vi "RLCar_joystick.vi"() -> ()   [LabVIEW 2021]
uses:
  Ctrl/joystick cfg.ctl
  Ctrl/joy-axis.ctl
  Ctrl/cmd_common.ctl
  <vilib>/Instr/_visa.llb/VISA Configure Serial Port (Instr).vi
  Log/_common_log/logfile-name.vi
panel:
  in  "Joystick cfg 2":T1={"steer limit"={"scale"=13.0, "offset"=32.0}, "speed limit"={"min"=10.0, "max"=161.0}, "Axis"={"man"=0.0, "auto"=0.0, "angular"=enum."Z rotation", "linear"=enum."X axis", "linear inv"=TRUE, "ang inv"=FALSE}} {"speed limit"."max" min=0.0 max=254.0 step=1.0}
  out "log path":string="C:\\RLmodel_cfg\\Log\\RLRobot\\2024-01-17-957\\Log_20240117-0957.txt"
  out "pos str":string="0"
  out "sp":dbl
  out "st":dbl=25.0 format="%.1f"
  out "val check":bool
  out "cmd_vel":cluster{dbl, dbl} {"?" format="%#.1f"; "?" format="%.1f"}
  out "n":i32=110
  out "XY Graph":cluster{cluster{"X":dbl, "Y":dbl}[]}[](graph)
  out "error out":errorcluster={"status"=FALSE, "code"=1073676294, "source"="VISA Read in RLCar_joystick.vi"}
  in  "port":refnum<visa-resource-name>="COM20"
  in  "rate":u32=115200
  out "Status":string
  out "String":string="sp=0,st=25,dir=b,light=1,pos=0,&\r\n"
  out "write buffer":string="0,25,b,1,RLCar kit ., &"
  in  "Led":bool=TRUE
  in  "msg":string="RLCar kit "
  in  "Write":bool=TRUE
  out "seriai buff":u32(graph)=34
  out "N":i32=221
  out "read buffer":string="sp=0,st=25,dir=b,light=1,pos=0,&\r\n"
  out "read buffer 2":string="sp=0,st=25,dir=b,light=1,pos=0,&\r\n"
  out "seriai R feedback":i32(graph)
  out "speed":dbl(graph)
  out "pos int":i32
  in  "dt":u32=50
  out "Recovery":i32
  in  "stop":bool=TRUE
  # "RLCar joystick controll"
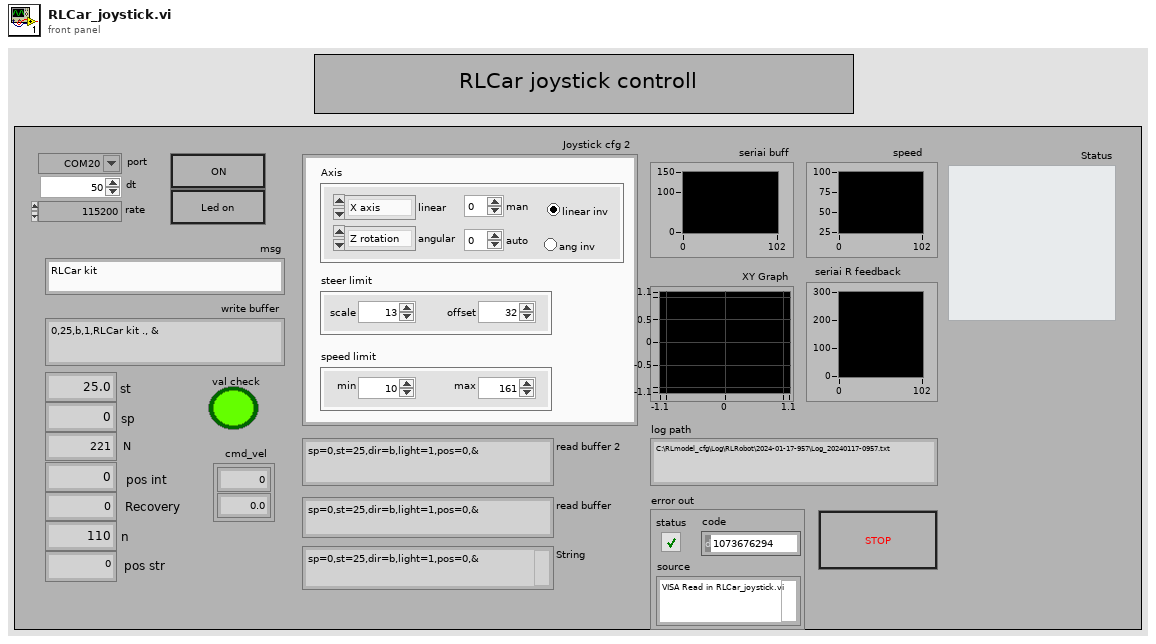
[diagram p1: front panel]
types:
  T1 = typedef "joystick cfg.ctl" = cluster{"steer limit":cluster{"scale":dbl, "offset":dbl}, "speed limit":cluster{"min":dbl, "max":dbl}, "Axis":cluster{"man":dbl, "auto":dbl, "angular":T2, "linear":T2, "linear inv":bool, "ang inv":bool}}
  T2 = typedef "joy-axis.ctl" = enum16{"X axis", "Y axis", "Z axis", "X rotation", "Y rotation", "Z rotation", "U axis", "V axis"}
  T3 = cluster{"axis info":cluster{"X axis":i32, "Y axis":i32, "Z axis":i32, "X axis rotation":i32, "Y axis rotation":i32, "Z axis rotation":i32, "U axis":i32, "V axis":i32}, "button info":cluster{"button 1":bool, "button 2":bool, "button 3":bool, "button 4":bool, "button 5":bool, "button 6":bool, "button 7":bool, "button 8":bool, "button 9":bool, "button 10":bool, "button 11":bool, "button 12":bool, "button 13":bool, "button 14":bool, "button 15":bool, "button 16":bool, "button 17":bool, "button 18":bool, "button 19":bool, "button 20":bool, "button 21":bool, "button 22":bool, "button 23":bool, "button 24":bool, "button 25":bool, "button 26":bool, "button 27":bool, "button 28":bool, "button 29":bool, "button 30":bool, "button 31":bool, "button 32":bool}, "direction info":cluster{"pov 1":i32, "pov 2":i32, "pov 3":i32, "pov 4":i32}}
  T4 = typedef "cmd_common.ctl" = enum16{"read", "write"}
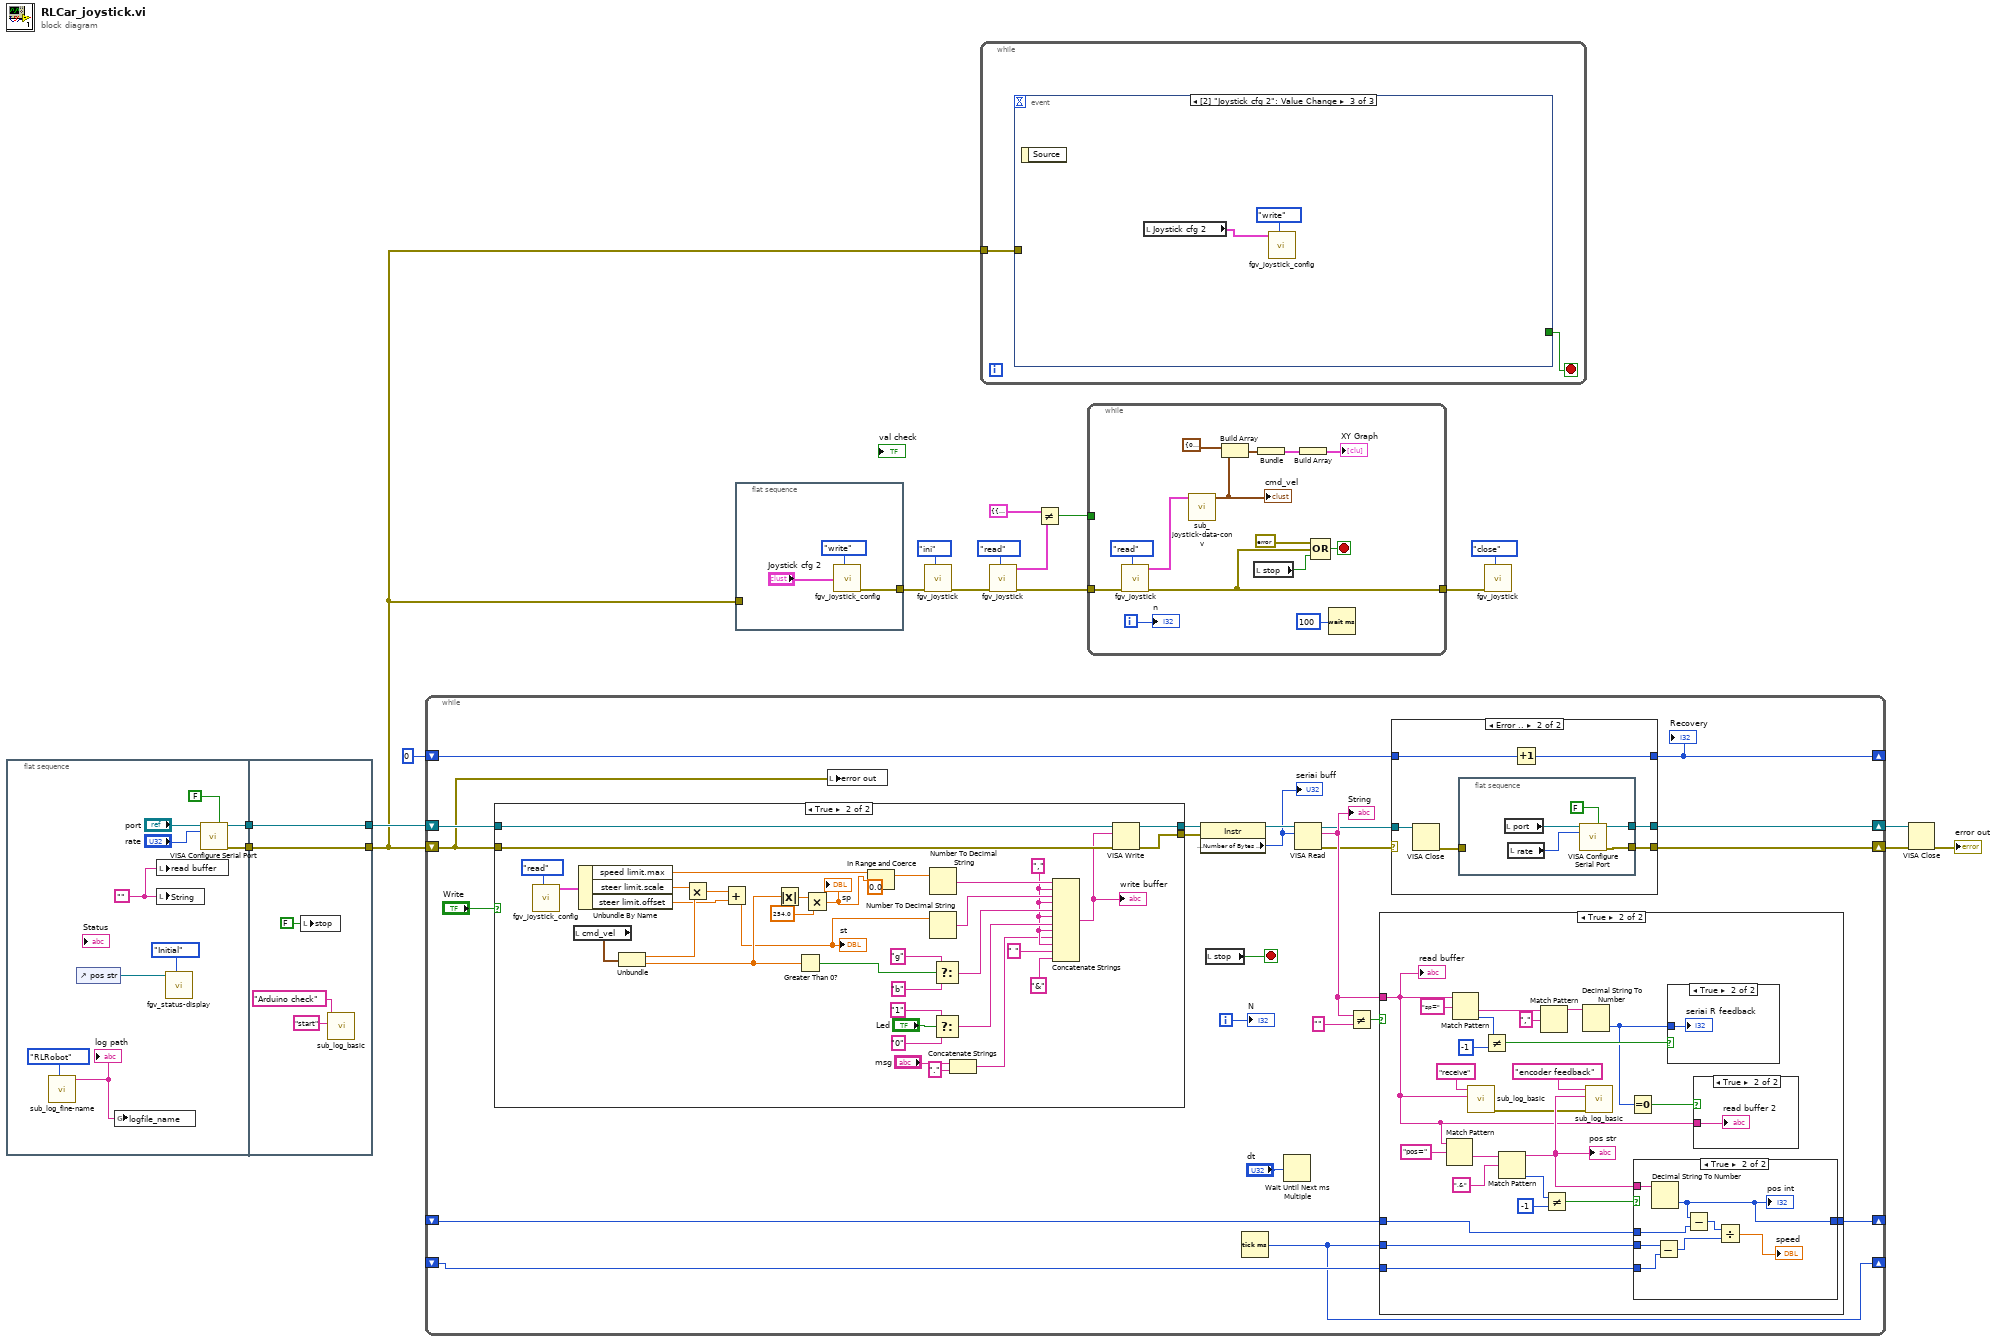
[diagram p0: block diagram]
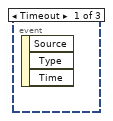
[diagram p2: hidden frame]
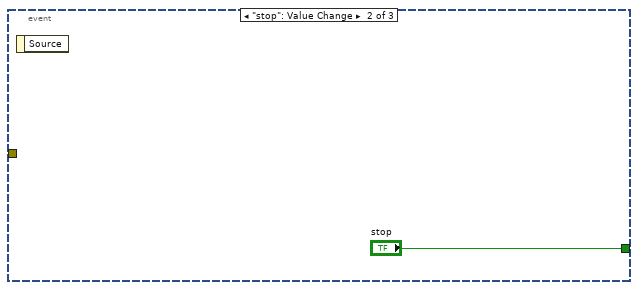
[diagram p3: hidden frame]
diagram:
  n1 = flat-sequence {
    tunnel: [w27] -> w18
    tunnel: [w26] -> w17
    tunnel: [w32] -> w1
    tunnel: [w33] -> w16
    tunnel: w18 -> [w33]
    tunnel: w17 -> [w32]
    frame #0 {
      w23 = ""
      n2 = call "sub_log_fine-name.vi"("Sel"=enum16{"RLRobot", "RLGPS"}."RLRobot") -> ("log path"=w19:string)  [unwired: 10 in]
      "log path" <- w19
      n3 = control-ref of="pos str"() -> (w21:refnum<vi>)
      n4 = global write "logfile-name.vi" "logfile_name"(w19) -> ()
      n5 = local write "read buffer"(w23) -> ()
      n6 = local write "String"(w23) -> ()
      n7 = call "fgv_status-display.vi"("Mode"=enum16{"Initial", "Update", "Clear"}."Initial", "System Log"=w21) -> ()  [unwired: 9 in, 1 out]
      n8 = call-poly "VISA Configure Serial Port"("port"="port", "Enable Termination\nChar (T)"=FALSE ("Enable Termination\nChar (T)"), "baud rate (9600)"="rate") -> ("port out"=w27:refnum<visa-resource-name>, "error out"=w26:errorcluster)  [unwired: 11 in]
    }
    frame #1 {
      n9 = local write "stop"(FALSE ("stop")) -> ()
      n10 = call "sub_log_basic.vi"("desc"="start", "Title"="Arduino check") -> ()  [unwired: 9 in, 1 out]
    }
  }
  n11 = while {
    shift-right: [w42] -> w15
    shift-left: w16 -> [w56]
    shift-right: [w43] -> w14
    shift-left: w1 -> [w39]
    shift-right: [w40] -> _
    shift-left: 0 -> [w41]
    shift-right: [w37] -> _
    shift-left: _ -> [w38]
    shift-right: [w36] -> _
    shift-left: _ -> [w35]
    i -> [w50]
    stop <- w34 stop-if-true
    n12 = case shown="True" "Write" {
      tunnel: w56 -> [w108 w144]
      tunnel: [w107 w143] -> w51
      tunnel: w39 -> [w107 w142]
      tunnel: [w108 w141] -> w53
      frame False {
      }
      frame True {
        w130 = "," ("string")
        n13 = call "fgv_joystick_config.vi"("cmd"=cmd_common."read") -> ("Joystick cfg 3"=w118:T1)  [unwired: 9 in, 1 out]
        n14 = local read "cmd_vel"() -> (w124:cluster{dbl, dbl})
        n15 = Unbundle By Name(w118) -> ("speed limit.max"=w114:dbl, "steer limit.scale"=w113:dbl, "steer limit.offset"=w110:dbl)
        n16 = Unbundle(w124) -> (w112:dbl, w122:dbl)
        n17 = Multiply(x=w113, y=w112) -> (x*y=w111:dbl)
        n18 = Add(x=w111, y=w110) -> (x+y=w109:dbl)
        "st" <- w109
        n19 = Absolute Value(x=w122) -> (abs(x)=w121:dbl)
        n20 = Greater Than 0?(x=w122) -> (x > 0?=w123:bool)
        n21 = Multiply(x=w121, y=254.0) -> (x*y=w116:dbl)
        "sp" <- w116
        n22 = In Range and Coerce(upper limit=w114, x=w116, lower limit=0.0) -> (coerced(x)=w115:dbl)  [unwired: 1 out]
        n23 = Number To Decimal String(number=w115) -> (decimal integer string=w140:string)  [unwired: 1 in]
        n24 = Number To Decimal String(number=w109) -> (decimal integer string=w138:string)  [unwired: 1 in]
        n25 = Select(t="g" ("string"), s=w123, f="b" ("string")) -> (s? t:f=w135:string)
        n26 = Select(t="1" ("string"), s="Led", f="0" ("string")) -> (s? t:f=w131:string)
        n27 = Concatenate Strings("msg", "." ("string")) -> (w127:string)
        n28 = Concatenate Strings(w140, w130, w138, w130, w135, w130, w131, w130, w127, w130, " " ("문자열"), "&" ("string")) -> (w125:string)
        "write buffer" <- w125
        n29 = VISA Write(VISA resource name=w144, write buffer=w125, error in (no error)=w142) -> (VISA resource name out=w141:refnum<visa-resource-name>, error out=w143:errorcluster)  [unwired: 1 out]
      }
    }
    n30 = local write "error out"(w39) -> ()
    n31 = property class="Instr"(reference=w53, error in=w51) -> (reference out=w54:refnum<visa-resource-name>, "Serial Settings:Number of Bytes at Serial Port"=w49:u32)  [unwired: 1 out]
    "seriai buff" <- w49
    n32 = local read "stop"() -> (w34:bool)
    n33 = Tick Count (ms)() -> (millisecond timer value=w37:u32)
    n34 = Wait Until Next ms Multiple(millisecond multiple="dt") -> ()  [unwired: 1 out]
    n35 = VISA Read(VISA resource name=w54, byte count=w49) -> (VISA resource name out=w44:refnum<visa-resource-name>, read buffer=w46:string, error out=w45:errorcluster)  [unwired: 1 in, 1 out]
    "String" <- w46
    n36 = Not Equal?(x=w46, y="") -> (x != y?=w47:bool)
    n37 = case shown="True" w47 {
      tunnel: w46 -> [_ w73]
      tunnel: w38 -> [_ w80]
      tunnel: w37 -> [_ w79]
      tunnel: [w71 w78] -> w36
      tunnel: w35 -> [w71 w77]
      frame False {
      }
      frame True {
        n38 = Match Pattern(string=w73, regular expression="pos=" ("정규식")) -> (after substring=w84:string)  [unwired: 1 in, 3 out]
        n39 = Match Pattern(string=w73, regular expression="sp=" ("정규식")) -> (after substring=w92:string, offset past match=w90:i32)  [unwired: 1 in, 2 out]
        n40 = call "sub_log_basic.vi"("desc"=w73, "Title"="receive") -> ("error out"=w72:errorcluster)  [unwired: 9 in]
        n41 = Not Equal?(x=w90, y=-1) -> (x != y?=w88:bool)
        n42 = Match Pattern(string=w84, regular expression=",&") -> (before substring=w75:string, offset past match=w82:i32)  [unwired: 1 in, 2 out]
        "pos str" <- w75
        n43 = Match Pattern(string=w92, regular expression="," ("정규식")) -> (before substring=w93:string)  [unwired: 1 in, 3 out]
        n44 = Not Equal?(x=w82, y=-1) -> (x != y?=w81:bool)
        n45 = Decimal String To Number(string=w93) -> (number=w87:i32)  [unwired: 2 in, 1 out]
        n46 = call "sub_log_basic.vi"("error in"=w72, "desc"=w75, "Title"="encoder feedback") -> ()  [unwired: 8 in, 1 out]
        n47 = Equal To 0?(x=w87) -> (x = 0?=w91:bool)
        n48 = case shown="True" w81 {
          tunnel: w75 -> [_ w104]
          tunnel: w80 -> [_ w102]
          tunnel: w79 -> [_ w103]
          tunnel: [w96 w99] -> w78
          tunnel: w77 -> [w96 w98]
          frame False {
          }
          frame True {
            n49 = Decimal String To Number(string=w104) -> (number=w99:i32)  [unwired: 2 in, 1 out]
            "pos int" <- w99
            n50 = Subtract(x=w103, y=w102) -> (x-y=w101:u32)
            n51 = Subtract(x=w99, y=w98) -> (x-y=w97:i32)
            n52 = Divide(x=w97, y=w101) -> (x/y=→"speed":dbl)
          }
        }
        n53 = case shown="True" w88 {
          tunnel: w87 -> [_ w105]
          frame False {
          }
          frame True {
            "seriai R feedback" <- w105
          }
        }
        n54 = case shown="True" w91 {
          tunnel: w73 -> [_ w106]
          frame False {
          }
          frame True {
            "read buffer 2" <- w106
          }
        }
        "read buffer" <- w73
      }
    }
    n55 = case shown="Error .." w45 {
      selector: w45 -> [w58 _]
      tunnel: w44 -> [w59 w65]
      tunnel: [w58 w63] -> w43
      tunnel: [w59 w62] -> w42
      tunnel: w41 -> [w57 w61]
      tunnel: [w57 w60] -> w40
      frame No Error {
      }
      frame Error {
        n56 = VISA Close(VISA resource name=w65) -> (error out=w64:errorcluster)  [unwired: 1 in]
        n57 = flat-sequence {
          tunnel: w64 -> [_]
          tunnel: [w67] -> w63
          tunnel: [w66] -> w62
          frame #0 {
            n58 = local read "port"() -> (w69:refnum<visa-resource-name>)
            n59 = local read "rate"() -> (w68:u32)
            n60 = call-poly "VISA Configure Serial Port"("port"=w69, "Enable Termination\nChar (T)"=FALSE ("Enable Termination\nChar (T)"), "baud rate (9600)"=w68) -> ("port out"=w66:refnum<visa-resource-name>, "error out"=w67:errorcluster)  [unwired: 11 in]
          }
        }
        n61 = Increment(x=w61) -> (x+1=w60:i32)
      }
    }
    "Recovery" <- w40
    "N" <- w50
  }
  n62 = flat-sequence {
    tunnel: [w146] -> w2
    tunnel: w1 -> [_]
    frame #0 {
      n63 = call "fgv_joystick_config.vi"("cmd"=cmd_common."write", "Joystick cfg 2"="Joystick cfg 2") -> ("error out"=w146:errorcluster)  [unwired: 8 in, 1 out]
    }
  }
  n64 = call "fgv_joystick.vi"("cmd"=enum16{"ini", "read", "close"}."ini", "error in"=w2) -> ("error out"=w7:errorcluster)  [unwired: 7 in, 2 out]
  n65 = while {
    tunnel: w1 -> [w149]
    stop <- w148 stop-if-true
    n66 = event shown="[2] \"Joystick cfg 2\": Value Change" {
      selector: _ -> [_ _ _]
      dyn-events: _ -> [_ _ _]
      timeout: _ -> [_ _ _]
      tunnel: w149 -> [_ _ _]
      tunnel: [_ "stop" _] -> w148
      event Timeout {
        n67 = event-data() -> ()  [unwired: 1 in, 3 out]
      }
      event "stop": Value Change {
        n68 = event-data() -> ()  [unwired: 1 in, 1 out]
      }
      event Value Change {
        n69 = event-data() -> ()  [unwired: 1 in, 1 out]
        n70 = local read "Joystick cfg 2"() -> (w151:T1)
        n71 = call "fgv_joystick_config.vi"("cmd"=cmd_common."write", "Joystick cfg 2"=w151) -> ()  [unwired: 8 in, 2 out]
      }
    }
  }
  n72 = call "fgv_joystick.vi"("cmd"=enum16{"ini", "read", "close"}."read", "error in"=w7) -> ("error out"=w6:errorcluster, "joystick info-out"=w4:T3)  [unwired: 7 in, 1 out]
  n73 = Not Equal?(x=T3 {"axis info"={"X axis"=0, "Y axis"=-256, "Z axis"=0, "X axis rotation"=0, "Y axis rotation"=0, "Z axis rotation"=-256, "U axis"=0, "V axis"=0}, "button info"={"button 1"=FALSE, "button 2"=FALSE, "button 3"=FALSE, "button 4"=FALSE, "button 5"=FALSE, "button 6"=FALSE, "button 7"=FALSE, "button 8"=FALSE, "button 9"=FALSE, "button 10"=FALSE, "button 11"=FALSE, "button 12"=FALSE, "button 13"=FALSE, "button 14"=FALSE, "button 15"=FALSE, "button 16"=FALSE, "button 17"=FALSE, "button 18"=FALSE, "button 19"=FALSE, "button 20"=FALSE, "button 21"=FALSE, "button 22"=FALSE, "button 23"=FALSE, "button 24"=FALSE, "button 25"=FALSE, "button 26"=FALSE, "button 27"=FALSE, "button 28"=FALSE, "button 29"=FALSE, "button 30"=FALSE, "button 31"=FALSE, "button 32"=FALSE}, "direction info"={"pov 1"=-1, "pov 2"=-1, "pov 3"=-1, "pov 4"=-1}} ("joystick info-out 2"), y=w4) -> (x != y?=w3:bool)
  n74 = while {
    tunnel: [w163] -> w9
    tunnel: w6 -> [w164]
    tunnel: w3 -> [_]
    i -> [w161]
    stop <- w162 stop-if-true
    n75 = call "fgv_joystick.vi"("cmd"=enum16{"ini", "read", "close"}."read", "error in"=w164) -> ("error out"=w163:errorcluster, "joystick info-out"=w155:T3)  [unwired: 7 in, 1 out]
    n76 = call "sub_joystick-data-conv.vi"("joystick info-in"=w155) -> ("opval"=w154:cluster{dbl, dbl})  [unwired: 9 in, 1 out]
    "cmd_vel" <- w154
    n77 = Build Array(cluster{"X":dbl, "Y":dbl} {"X"=0.0, "Y"=0.0}, w154) -> (w159:cluster{"X":dbl, "Y":dbl}[])
    n78 = local read "stop"() -> (w153:bool)
    n79 = Bundle(w159) -> (w158:cluster{cluster{"X":dbl, "Y":dbl}[]})  [unwired: 1 in]
    n80 = Build Array(w158) -> (→"XY Graph":cluster{cluster{"X":dbl, "Y":dbl}[]}[])
    n81 = Compound Arithmetic op=OR(errorcluster {"status"=FALSE, "code"=0, "source"=""} ("value"), w163, w153) -> (w162:bool)
    n82 = Wait (ms)(milliseconds to wait=u32 100) -> ()  [unwired: 1 out]
    "n" <- w161
  }
  n83 = call "fgv_joystick.vi"("cmd"=enum16{"ini", "read", "close"}."close", "error in"=w9) -> ()  [unwired: 7 in, 3 out]
  n84 = VISA Close(VISA resource name=w15, error in (no error)=w14) -> (error out=→"error out":errorcluster)
